vi "benchmark of to 1d array.vi"() -> ()   [LabVIEW 2017]
uses:
  <userlib>/_NEVSTOP/Communicable State Machine(CSM)/Communicable State Machine.lvlib
  addons/API-String-Arugments-Support/API String Arguments Support.lvlib
panel:
  out "Numeric 2":dbl format="%#_6p"
  out "Array of Strings 2":string[](array[string])
  out "Array of Strings":string[](array[string])
  out "Numeric":dbl format="%#_6p"
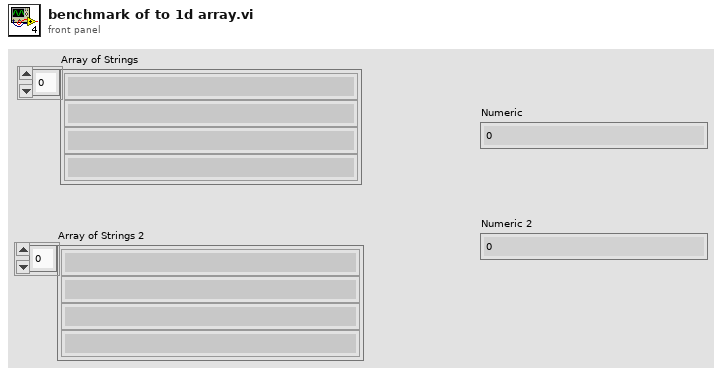
[diagram p1: front panel]
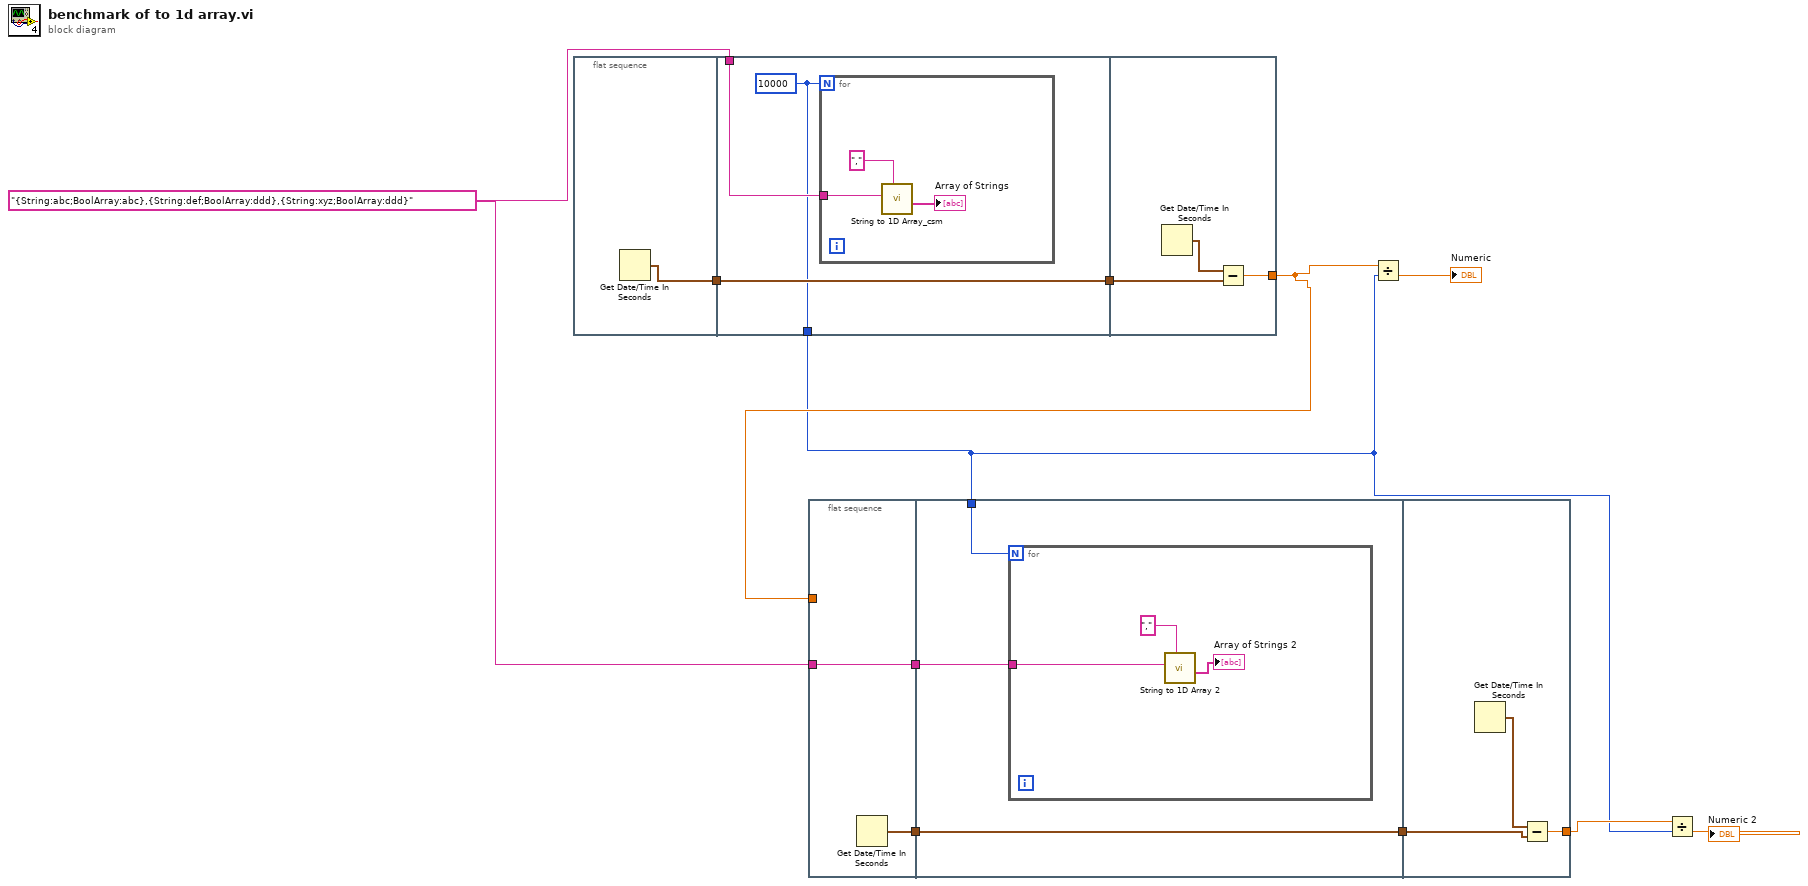
[diagram p0: block diagram]
diagram:
  w11 = "{String:abc;BoolArray:abc},{String:def;BoolArray:ddd},{String:xyz;BoolArray:ddd}" ("String")
  n1 = flat-sequence {
    tunnel: [w12] -> w10
    tunnel: w11 -> [w15]
    tunnel: w10 -> [w14]
    tunnel: [w14] -> w9
    tunnel: [w13] -> w1
    tunnel: w9 -> [w20]
    tunnel: [w19] -> w3
    frame #0 {
      n2 = Get Date/Time In Seconds() -> (seconds since 1Jan1904=w12:timestamp)
    }
    frame #1 {
      w13 = 10000
      n3 = for {
        N: w13 -> [_]
        tunnel: w15 -> [w17]
        n4 = call <userlib>:"String to 1D Array_csm.vi"("delimiter (Tab)"=",", "string"=w17) -> ("Array of Strings"=→"Array of Strings":string[])  [unwired: 9 in]
      }
    }
    frame #2 {
      n5 = Get Date/Time In Seconds() -> (seconds since 1Jan1904=w21:timestamp)
      n6 = Subtract(x=w21, y=w20) -> (x-y=w19:dbl)
    }
  }
  n7 = flat-sequence {
    tunnel: w11 -> [w23]
    tunnel: [w23] -> w8
    tunnel: [w22] -> w7
    tunnel: w3 -> [_]
    tunnel: w8 -> [w26]
    tunnel: w7 -> [w25]
    tunnel: [w25] -> w6
    tunnel: w1 -> [w24]
    tunnel: w6 -> [w31]
    tunnel: [w30] -> w2
    frame #0 {
      n8 = Get Date/Time In Seconds() -> (seconds since 1Jan1904=w22:timestamp)
    }
    frame #1 {
      n9 = for {
        N: w24 -> [_]
        tunnel: w26 -> [w29]
        n10 = call "String to 1D Array 2.vi"("delimiter (,)"=",", "string"=w29) -> ("Array of Strings"=→"Array of Strings 2":string[])  [unwired: 8 in, 1 out]
      }
    }
    frame #2 {
      n11 = Get Date/Time In Seconds() -> (seconds since 1Jan1904=w32:timestamp)
      n12 = Subtract(x=w32, y=w31) -> (x-y=w30:dbl)
    }
  }
  n13 = Divide(x=w3, y=w1) -> (x/y=→"Numeric":dbl)
  n14 = Divide(x=w2, y=w1) -> (x/y=→"Numeric 2":dbl)
